vi "set_parameter.vi"(6 "timeout (25000ms)":i32=25000, 8 "error in (no error)":errorcluster, 9 "values":dbl[](array[numeric]), 10 "set parameters":T1[](array[typedef]), 11 "daemon reference in":refnum<k5>) -> (0 "error out":errorcluster, 2 "response":string, 3 "daemon reference out":refnum<k5>, 5 "command out":string="random")   [LabVIEW 2017]
doc: "<b>Command: </b>\"set_parameter\"\n\n<b>Description: </b> Instructs the target to set the specified parameter values.\n\n<b>Parameters: </b> \n\n 1. Parameter Array [max 20]\n 2. Value Array\n____________________________________________\nDIPC 692 Daemon API 10.0.0.1\nSam Tee - Dyson Technology Ltd\nCopyright (c) 2024, Dyson Technology Ltd"
uses:
  typdef/set_parameter.ctl
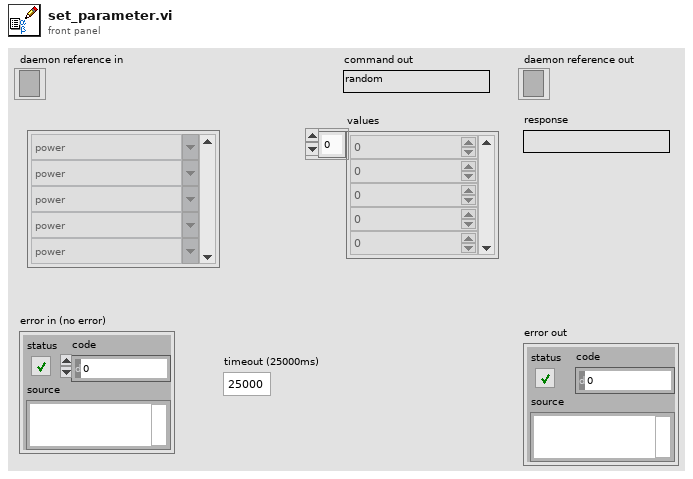
[diagram p1: front panel]
types:
  T1 = typedef "set_parameter.ctl" = string
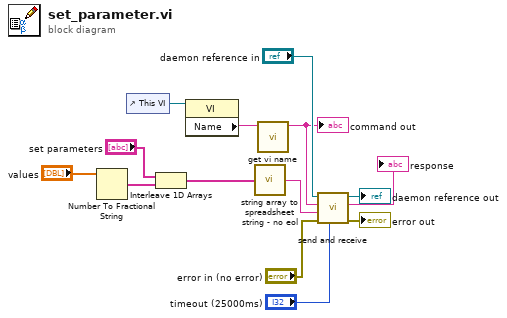
[diagram p0: block diagram]
diagram:
  n1 = Number To Fractional String(number="values") -> (F-format string=w4:string[])  [unwired: 3 in]
  n2 = control-ref of="This VI"() -> (w9:refnum<vi>)
  n3 = Interleave 1D Arrays("set parameters", w4) -> (w1:T1[])
  n4 = property class="VI"(reference=w9) -> ("Name"=w8:string)  [unwired: 1 in, 2 out]
  n5 = call "string array to spreadsheet string - no eol.vi"("string array"=w1) -> ("spreadsheet string - no eol"=w3:string)
  n6 = call "get vi name.vi"("library.lvlib:name.vi"=w8) -> ("vi name"=w7:string)  [unwired: 10 in]
  "command out" <- w7
  n7 = call "send and receive.vi"("timeout (25000ms)"="timeout (25000ms)", "error in (no error)"="error in (no error)", "data"=w3, "command"=w7, "daemon reference in"="daemon reference in") -> ("error out"=→"error out":errorcluster, "response"=→"response":string, "daemon reference out"=→"daemon reference out":refnum<k5>)  [unwired: 4 in]
